vi "NI DAQ init.vi"(7 "trigger frequency":dbl format="%#_13g", 8 "error in":errorcluster, 11 "DAQmx Device Name":tag="PXI2Slot6") -> (0 "error out":errorcluster, 3 "DAQmx Device Name Out":tag="PXI2Slot6")   [LabVIEW 2020]
uses:
  <vilib>/DAQmx/write.llb/DAQmx Write (Analog 1D DBL 1Chan NSamp).vi
  NI DAQ globals.vi
  <vilib>/DAQmx/create/channels.llb/DAQmx Create Channel (CO-Pulse Generation-Frequency).vi
  <vilib>/DAQmx/configure/timing.llb/DAQmx Timing (Implicit).vi
  <vilib>/DAQmx/create/channels.llb/DAQmx Create Channel (AO-Voltage-Basic).vi
  <vilib>/DAQmx/configure/timing.llb/DAQmx Timing (Sample Clock).vi
  <vilib>/DAQmx/miscellaneous.llb/DAQmx Fill In Error Info.vi
  <resource>/objmgr/daqmx.rc
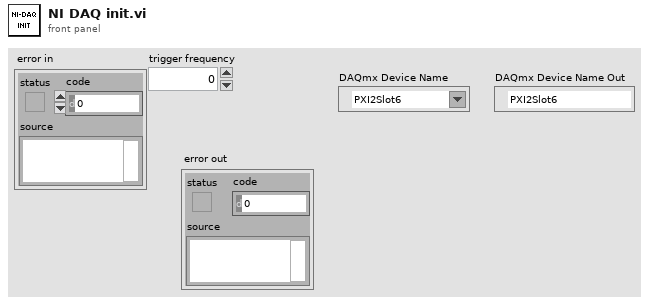
[diagram p1: front panel]
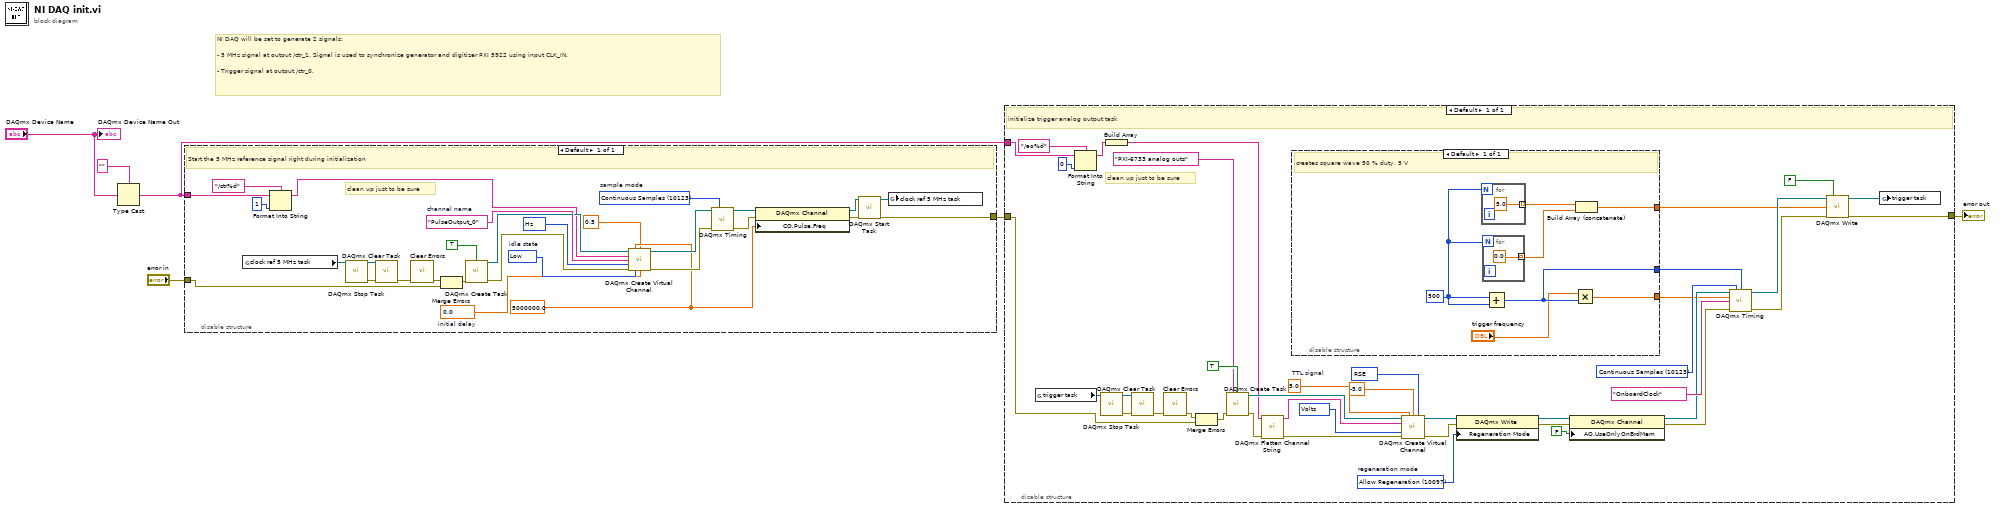
[diagram p0: block diagram]
diagram:
  # "NI DAQ will be set to generate 2 signals:\n\n- 5 MHz signal at output /ctr_1. Signal is used to synchronize generator and digitizer PXI 5922 using input CLK_IN.\n\n- Trigger signal at output /ctr_0."
  n1 = Type Cast(type="", x="DAQmx Device Name") -> (*(type *) &x=w3:string)
  n2 = disable-structure shown="Default" {
    disable-tunnel: "error in" -> [w9]
    disable-tunnel: [w15] -> w2
    disable-tunnel: w3 -> [w14]
    frame Enabled {
      w27 = 10373 items=["Hz"=10373] ("units")
      w31 = 5000000.0 ("frequency")
      w30 = 10123 items=["Finite Samples"=10178, "Continuous Samples"=10123, "Hardware Timed Single Point"=12522]  # sample mode
      w25 = 0.0  # initial delay
      w26 = 10214 items=["High"=10192, "Low"=10214]  # idle state
      w28 = "PulseOutput_0"  # channel name
      # "clean up just to be sure"
      # "Start the 5 MHz reference signal right during initialization"
      n3 = global read "NI DAQ globals.vi" "clock ref 5 MHz task"() -> (w10:refnum<k21>)
      n4 = Format Into String(format string="/ctr%d", initial string=w14, 1 ("input 1")) -> (resulting string=w17:string)  [unwired: 1 in, 1 out]
      n5 = call <vilib>:"DAQmx Stop Task.vi"("task/channels in"=w10) -> ("task out"=w13:refnum<k21>, "error out"=w12:errorcluster)  [unwired: 13 in]
      n6 = call <vilib>:"DAQmx Clear Task.vi"("task in"=w13, "error in"=w12) -> ("error out"=w11:errorcluster)  [unwired: 13 in]
      n7 = call <vilib>:"Clear Errors.vi"("error in (no error)"=w11) -> ("error out"=w8:errorcluster)  [unwired: 5 in, 1 out]
      n8 = Merge Errors(w8, w9) -> (w7:errorcluster)
      n9 = call <vilib>:"DAQmx Create Task.vi"("auto cleanup"=TRUE, "error in"=w7) -> ("task out"=w22:refnum<k21>, "error out"=w23:errorcluster)  [unwired: 12 in]
      n10 = call-poly <vilib>:"DAQmx Create Virtual Channel.vi"("task in"=w22, "frequency"=w31, "duty cycle"=0.5, "counter"=w17, "name to assign"=w28, "units"=w27, "error in"=w23, "idle state"=w26, "initial delay"=w25) -> ("task out"=w33:refnum<k21>, "error out"=w32:errorcluster)  [unwired: 5 in]
      n11 = call-poly <vilib>:"DAQmx Timing.vi"("task/channels in"=w33, "sample mode"=w30, "error in"=w32) -> ("task out"=w34:refnum<k21>, "error out"=w35:errorcluster)  [unwired: 11 in]
      n12 = property class="DAQmx Channel"(reference=w34, error in=w35, "CO.Pulse.Freq"=w31) -> (reference out=w20:refnum<k21>, error out=w21:errorcluster)
      n13 = call <vilib>:"DAQmx Start Task.vi"("task/channels in"=w20, "error in"=w21) -> ("task out"=w16:refnum<k21>, "error out"=w15:errorcluster)  [unwired: 12 in]
      n14 = global write "NI DAQ globals.vi" "clock ref 5 MHz task"(w16) -> ()
    }
  }
  n15 = disable-structure shown="Default" {
    disable-tunnel: w3 -> [w58]
    disable-tunnel: w2 -> [w39]
    disable-tunnel: [w44] -> w1
    frame Enabled {
      w49 = 10123 items=["Finite Samples"=10178, "Continuous Samples"=10123, "Hardware Timed Single Point"=12522] ("sample mode")
      w57 = 5.0  # TTL signal
      w68 = 10097 items=["Allow Regeneration"=10097, "Do Not Allow Regeneration"=10158]  # regeneration mode
      w69 = 10348 items=["Volts"=10348, "From Custom Scale"=10065] ("units")
      w70 = 10083 items=["Default"=-1, "RSE"=10083, "Differential"=10106, "Pseudodifferential"=12529] ("output terminal configuration")
      # "clean up just to be sure"
      # "initialize trigger analog output task"
      n16 = global read "NI DAQ globals.vi" "trigger task"() -> (w54:refnum<k21>)
      n17 = Format Into String(format string="/ao%d", initial string=w58, 0 ("input 1")) -> (resulting string=w60:string)  [unwired: 1 in, 1 out]
      n18 = call <vilib>:"DAQmx Stop Task.vi"("task/channels in"=w54) -> ("task out"=w55:refnum<k21>, "error out"=w53:errorcluster)  [unwired: 13 in]
      n19 = Build Array(w60) -> (w59:string[])
      n20 = call <vilib>:"DAQmx Clear Task.vi"("task in"=w55, "error in"=w53) -> ("error out"=w38:errorcluster)  [unwired: 13 in]
      n21 = call <vilib>:"Clear Errors.vi"("error in (no error)"=w38) -> ("error out"=w36:errorcluster)  [unwired: 5 in, 1 out]
      n22 = Merge Errors(w36, w39) -> (w37:errorcluster)
      n23 = call <vilib>:"DAQmx Create Task.vi"("new task name"="PXI-6733 analog outs", "auto cleanup"=TRUE, "error in"=w37) -> ("task out"=w74:refnum<k21>, "error out"=w73:errorcluster)  [unwired: 11 in]
      n24 = call <vilib>:"DAQmx Flatten Channel String.vi"("names in"=w59, "error in"=w73) -> ("names out"=w71:string, "error out"=w72:errorcluster)  [unwired: 12 in]
      n25 = disable-structure shown="Default" {
        disable-tunnel: [w82] -> w42
        disable-tunnel: [w81] -> w41
        disable-tunnel: [w78] -> w40
        frame Enabled {
          w76 = 500
          # "creates square wave 50 % duty, 5 V"
          n26 = for {
            N: w76 -> [_]
            tunnel: [5.0 ("rate")] -> w79 mode=indexing
          }
          n27 = for {
            N: w76 -> [_]
            tunnel: [0.0 ("rate")] -> w80 mode=indexing
          }
          n28 = Add(x=w76, y=w76) -> (x+y=w81:i32)
          n29 = Multiply(x="trigger frequency", y=w81) -> (x*y=w82:dbl)
          n30 = Build Array (concatenate)(w79, w80) -> (w78:dbl[])
        }
      }
      n31 = call-poly <vilib>:"DAQmx Create Virtual Channel.vi"("task in"=w74, "maximum value"=w57, "minimum value"=-5.0, "output terminal configuration"=w70, "physical channels"=w71, "units"=w69, "error in"=w72) -> ("task out"=w66:refnum<k21>, "error out"=w67:errorcluster)  [unwired: 7 in]
      n32 = property class="DAQmx Write"(reference=w66, error in=w67, "Regeneration Mode"=w68) -> (reference out=w63:refnum<k21>, error out=w64:errorcluster)
      n33 = property class="DAQmx Channel"(reference=w63, error in=w64, "AO.UseOnlyOnBrdMem"=FALSE) -> (reference out=w46:refnum<k21>, error out=w45:errorcluster)
      n34 = call-poly <vilib>:"DAQmx Timing.vi"("task/channels in"=w46, "sample mode"=w49, "samples per channel"=w41, "rate"=w42, "source"=tag "OnboardClock", "error in"=w45) -> ("task out"=w52:refnum<k21>, "error out"=w51:errorcluster)  [unwired: 8 in]
      n35 = call-poly <vilib>:"DAQmx Write.vi"("task/channels in"=w52, "auto start"=FALSE, "data"=w40, "error in"=w51) -> ("task out"=w47:refnum<k21>, "error out"=w44:errorcluster)  [unwired: 9 in, 1 out]
      n36 = global write "NI DAQ globals.vi" "trigger task"(w47) -> ()
    }
  }
  "error out" <- w1
  "DAQmx Device Name Out" <- "DAQmx Device Name"
